vi "Modbus GET SRI Array.vi"(8 "error in":errorcluster, 11 "Raw SRI Data in":string[](array[string])) -> (0 "error out":errorcluster, 3 "SRI Butane Levels":string[][](array[string]))   [LabVIEW 2020, in "Modbus.lvlib"]
uses:
  Modbus.lvlib
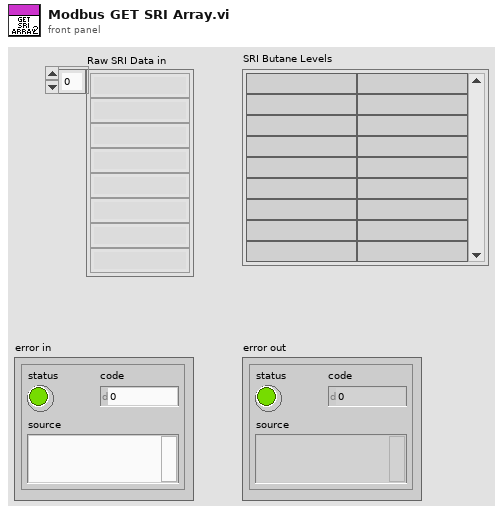
[diagram p1: front panel]
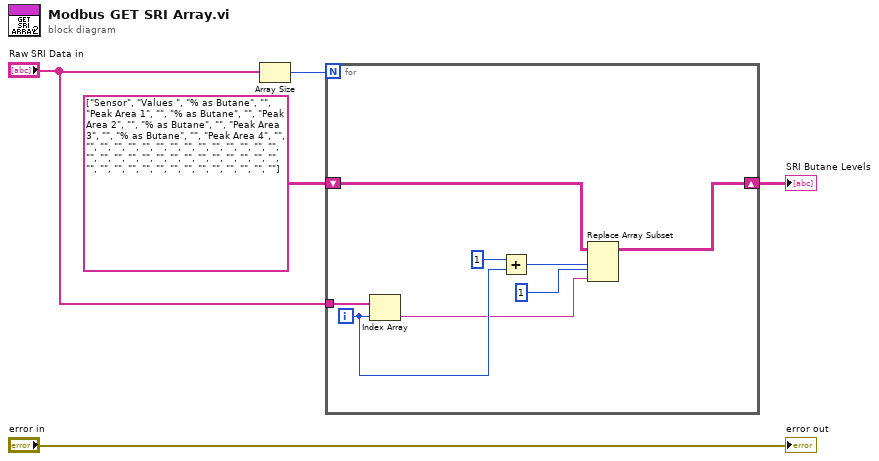
[diagram p0: block diagram]
diagram:
  n1 = Array Size(array="Raw SRI Data in") -> (size(s)=w3:i32)
  n2 = for {
    N: w3 -> [_]
    tunnel: "Raw SRI Data in" -> [w13]
    shift-right: [w6] -> w5
    shift-left: string[][] [["Sensor", "Values "], ["% as Butane", ""], ["Peak Area 1", ""], ["% as Butane", ""], ["Peak Area 2", ""], ["% as Butane", ""], ["Peak Area 3", ""], ["% as Butane", ""], ["Peak Area 4", ""], ["", ""], ["", ""], ["", ""], ["", ""], ["", ""], ["", ""], ["", ""], ["", ""], ["", ""], ["", ""], ["", ""], ["", ""], ["", ""], ["", ""], ["", ""], ["", ""], ["", ""], ["", ""], ["", ""], ["", ""], ["", ""]] ("Array 2") -> [w12]
    i -> [w9]
    n3 = Index Array(array=w13, index=w9) -> (element=w7:string)
    n4 = Add(x=1 ("disabled index (col)"), y=w9) -> (x+y=w11:i32)
    n5 = Replace Array Subset(array=w12, new element=w7, index (row)=w11, index (col)=1 ("disabled index (col)")) -> (w6:string[][])
  }
  "SRI Butane Levels" <- w5
  "error out" <- "error in"
